vi "Write Position.vi"(8 "error in (no error)":errorcluster, 10 "BC position 1D":T1 items=["Start X", "End X"], 11 "BC_Evolut_1D.lvclass in":refnum<class "NI_BC_Evolut_1D.lvclass">) -> (0 "error out":errorcluster, 3 "BC_Evolut_1D.lvclass out":refnum<class "NI_BC_Evolut_1D.lvclass">)   [LabVIEW 2020, in "NI_PDE.lvlib" / "NI_BC_Evolut_1D.lvclass"]
uses:
  <vilib>/gmath/pde.llb/BCClass/BC_Evolut_1D/NI_BC_Evolut_1D.lvclass
  <vilib>/gmath/pde.llb/Common/PDE_BC Position 1D.ctl
  <vilib>/gmath/pde.llb/BCClass/BC_Evolut_1D/NI_BC_Evolut_1D.lvclass/NI_BC_Evolut_1D.ctl
  <vilib>/gmath/NI_PDE.lvlib
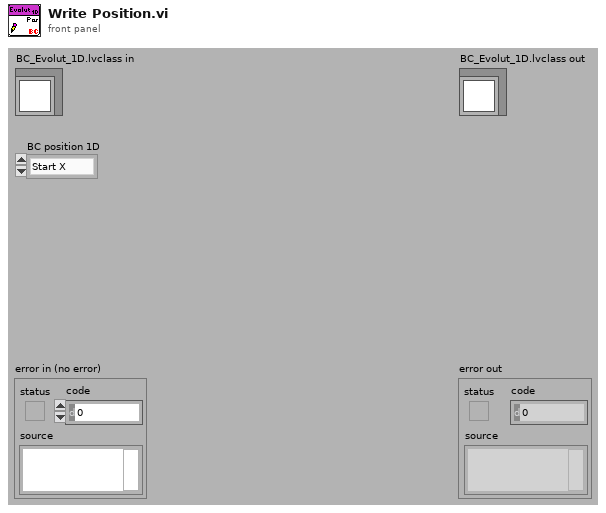
[diagram p1: front panel]
types:
  T1 = typedef "NI_PDE.lvlib/PDE_BC Position 1D.ctl" = i32
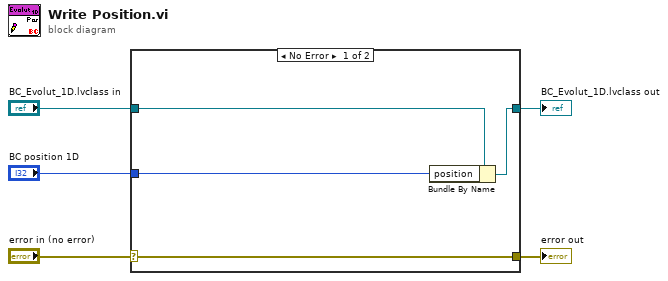
[diagram p0: block diagram]
diagram:
  n1 = case shown="No Error" "error in (no error)" {
    selector: "error in (no error)" -> [w9 w10]
    tunnel: [w9 w10] -> w4
    tunnel: [w7 w11] -> w2
    tunnel: "BC_Evolut_1D.lvclass in" -> [w8 w11]
    tunnel: "BC position 1D" -> [w6 _]
    frame No Error {
      n2 = Bundle By Name(cluster=w8, "position"=w6) -> (w7:refnum<class "NI_BC_Evolut_1D.lvclass">)
    }
    frame Error {
    }
  }
  "error out" <- w4
  "BC_Evolut_1D.lvclass out" <- w2
